vi "Test Server.vi"() -> ()   [LabVIEW 2013]
uses:
  <vilib>/LabVIEW Open Source Project/MQTT Control Packets/Control Packets/CONNACK/Connect Return Code -- enum.ctl
  Server/Server class/Server.lvclass/Server.ctl
  Client/Client Class/Client.lvclass/Client.ctl
  <vilib>/LabVIEW Open Source Project/MQTT Control Packets/Control Packets/PUBLISH/PUBLISH.lvclass
  Server/Server class/Server.lvclass
  MQTT_Base/Base Class/MQTT_Base.lvclass
  Client/Client Class/Client.lvclass
  MQTT_TCP/Connection/TCPConnection.lvclass
  <vilib>/LabVIEW Open Source Project/MQTT Control Packets/Control Packets/CONNACK/CONNACK.lvclass
panel:
  out "error server":errorcluster
  in  "Unsubscribe":bool
  in  "Subscribe":bool
  out "error client sink 2":errorcluster
  out "Random 2":dbl(graph)
  out "received 2":i32
  out "received timer 2":u32
  out "Client Status 2":T1=enum."Server Unavailable"
  out "published timer":u32
  out "received timer":u32
  out "received":i32
  out "published":i32
  out "Random":dbl(graph)
  out "Client Status":T1=enum."Server Unavailable"
  out "error client source":errorcluster
  out "NbConnections":u32
  out "error client sink 1":errorcluster
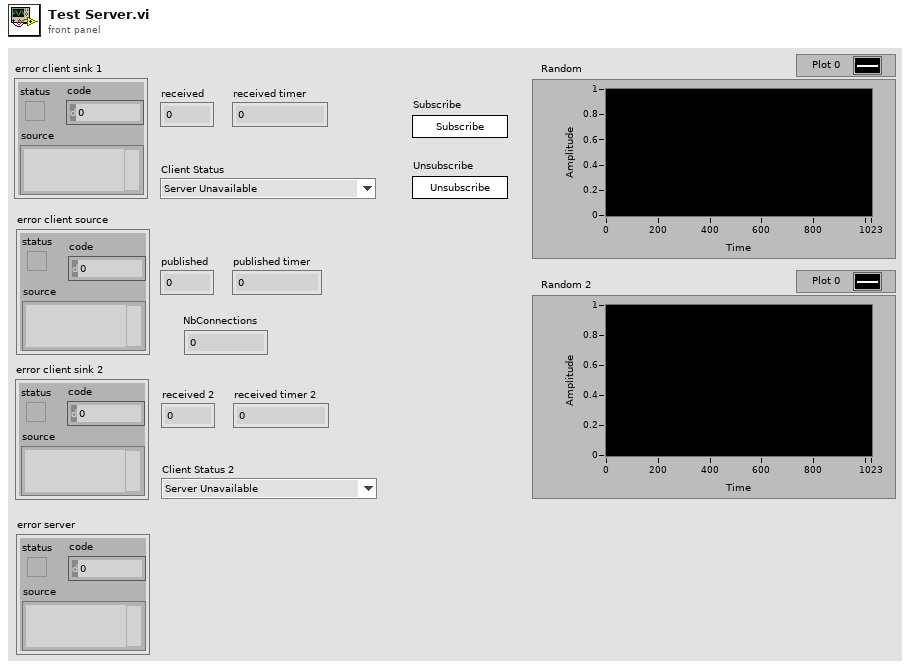
[diagram p1: front panel]
types:
  T1 = typedef "MQTT_Control_Packets.lvlib/CONNACK.lvclass/Connect Return Code -- enum.ctl" = enum16{"Connection accepted", "Unacceptable protocol version", "Identifier Rejected", "Server Unavailable", "Bad Username or Password", "Not Authorized"}
  T2 = typedef "MQTT Server.lvlib/Server.lvclass/Public Events -- cluster.ctl" = cluster{"NbConnections":refnum<user-event>}
  T3 = typedef "MQTT Client.lvlib/Client.lvclass/Public Events -- cluster.ctl" = cluster{"Connection Status":refnum<user-event>, "Connected":refnum<user-event>, "Application Message":refnum<user-event>}
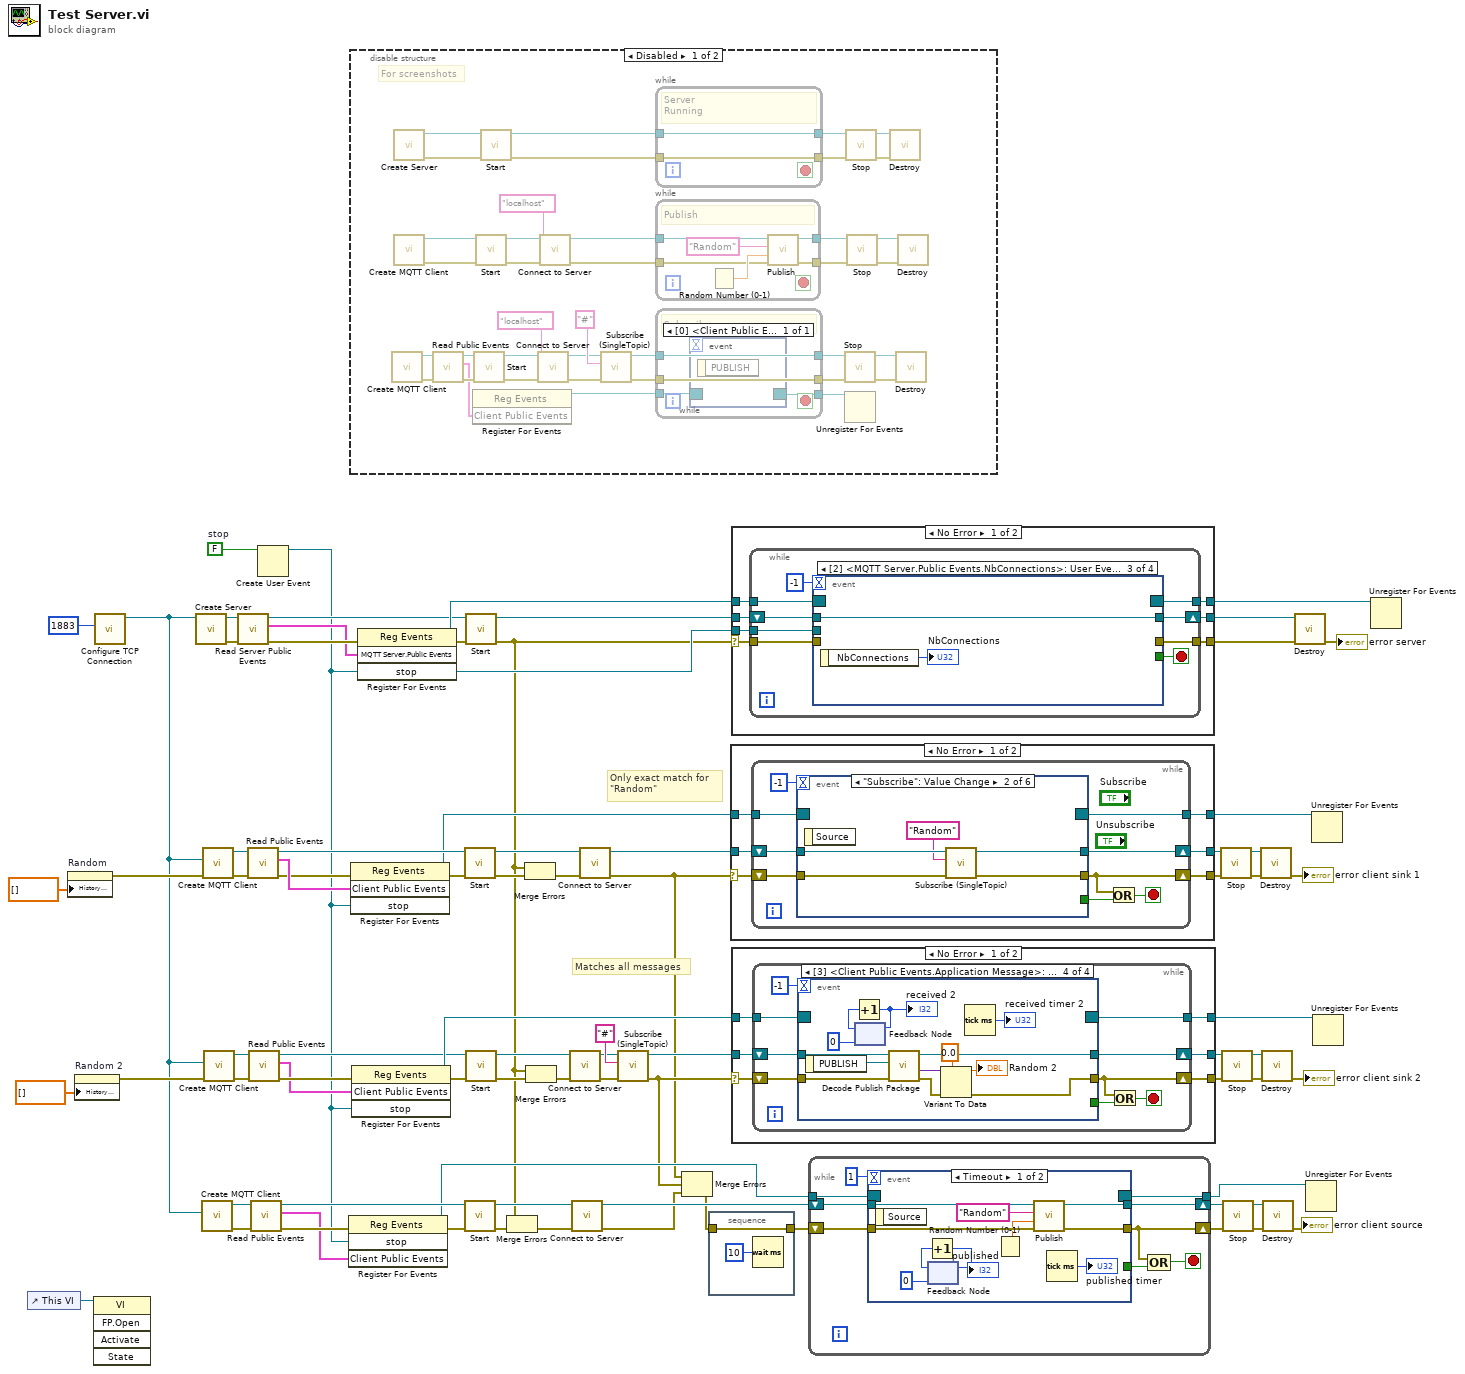
[diagram p0: block diagram]
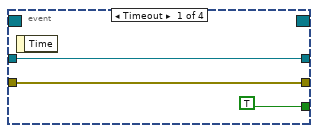
[diagram p3: hidden frame]
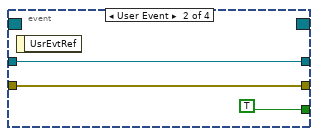
[diagram p4: hidden frame]
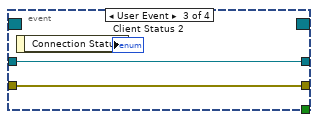
[diagram p5: hidden frame]
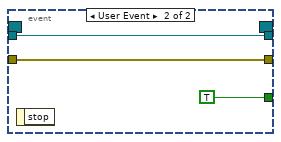
[diagram p7: hidden frame]
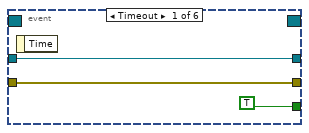
[diagram p8: hidden frame]
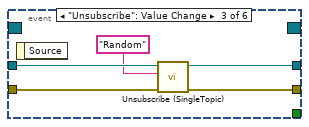
[diagram p9: hidden frame]
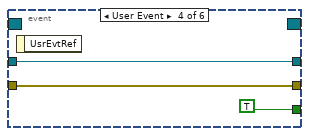
[diagram p10: hidden frame]
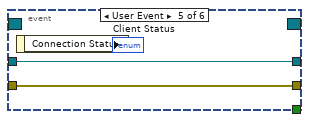
[diagram p11: hidden frame]
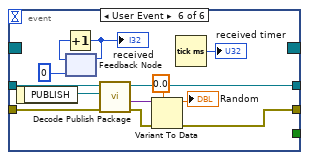
[diagram p12: hidden frame]
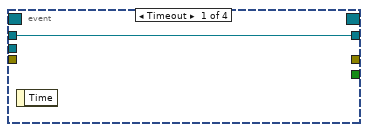
[diagram p14: hidden frame]
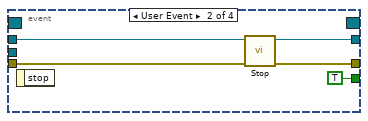
[diagram p15: hidden frame]
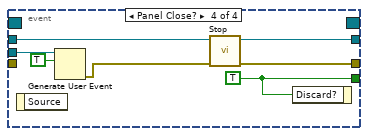
[diagram p16: hidden frame]
diagram:
  w39 = FALSE  # stop
  # "Matches all messages"
  # "Only exact match for\n\"Random\""
  n1 = control-ref of="This VI"() -> (w7:refnum<vi>)
  n2 = property on="Random" class="WFChart (strict)"("History Data"=dbl[] []) -> (error out=w43:errorcluster)  [unwired: 2 in, 1 out]
  n3 = property on="Random 2" class="WFChart (strict)"("History Data"=dbl[] []) -> (error out=w10:errorcluster)  [unwired: 2 in, 1 out]
  n4 = invoke class="VI" method="FP.Open"(reference=w7) -> ()  [unwired: 4 in, 5 out]
  n5 = call "Configure TCP Connection.vi"("remote port (80)"=u16 1883) -> ("TCPConnection"=w1:refnum<class "TCPConnection.lvclass">)  [unwired: 9 in, 1 out]
  n6 = call "Create Server.vi"("Connection Configuration"=w1) -> ("error out"=w79:errorcluster, "Server"=w80:refnum<class "Server.lvclass">)  [unwired: 9 in]
  n7 = call "Create MQTT Client.vi"("Connection Configuration"=w1) -> ("error out"=w63:errorcluster, "Client out"=w62:refnum<class "Client.lvclass">)  [unwired: 9 in]
  n8 = call "Create MQTT Client.vi"("error in (no error)"=w43, "Connection Configuration"=w1) -> ("error out"=w64:errorcluster, "Client out"=w65:refnum<class "Client.lvclass">)  [unwired: 8 in]
  n9 = call "Create MQTT Client.vi"("error in (no error)"=w10, "Connection Configuration"=w1) -> ("error out"=w15:errorcluster, "Client out"=w14:refnum<class "Client.lvclass">)  [unwired: 8 in]
  n10 = call "Read Server Public Events.vi"("error in (no error)"=w79, "Server in"=w80) -> ("error out"=w78:errorcluster, "MQTT Server.Public Events"=w77:T2, "Server out"=w73:refnum<class "Server.lvclass">)  [unwired: 7 in]
  n11 = call "Read Public Events.vi"("error in (no error)"=w64, "Client in"=w65) -> ("error out"=w48:errorcluster, "Client Public Events"=w49:T3, "Client out"=w61:refnum<class "Client.lvclass">)  [unwired: 7 in]
  n12 = call "Read Public Events.vi"("error in (no error)"=w15, "Client in"=w14) -> ("error out"=w26:errorcluster, "Client Public Events"=w25:T3, "Client out"=w16:refnum<class "Client.lvclass">)  [unwired: 7 in]
  n13 = call "Read Public Events.vi"("error in (no error)"=w63, "Client in"=w62) -> ("error out"=w38:errorcluster, "Client Public Events"=w34:T3, "Client out"=w58:refnum<class "Client.lvclass">)  [unwired: 7 in]
  n14 = Create User Event(user event datatype=w39) -> (user event=w11:refnum<user-event>)  [unwired: 1 in, 1 out]
  n15 = register-events(error in=w38, w11, w34) -> (reference out=w36:refnum<event-registration>, error out=w37:errorcluster)  [unwired: 1 in]
  n16 = disable-structure shown="Disabled" {
    frame Disabled {
      # "For screenshots"
      n17 = call "Create MQTT Client.vi"() -> ("error out"=w86:errorcluster, "Client out"=w88:refnum<class "Client.lvclass">)  [unwired: 10 in]
      n18 = call "Create Server.vi"() -> ("error out"=w113:errorcluster, "Server"=w112:refnum<class "Server.lvclass">)  [unwired: 10 in]
      n19 = call "Create MQTT Client.vi"() -> ("error out"=w110:errorcluster, "Client out"=w111:refnum<class "Client.lvclass">)  [unwired: 10 in]
      n20 = call "Read Public Events.vi"("error in (no error)"=w86, "Client in"=w88) -> ("error out"=w85:errorcluster, "Client Public Events"=w84:T3, "Client out"=w87:refnum<class "Client.lvclass">)  [unwired: 7 in]
      n21 = register-events(w84) -> (reference out=w83:refnum<event-registration>)  [unwired: 2 in, 1 out]
      n22 = call "Start.vi"("error in (no error)"=w85, "MQTT_Base in"=w87) -> ("error out"=w103:errorcluster, "MQTT_Base out"=w104:refnum<class "Client.lvclass">)  [unwired: 7 in, 1 out]
      n23 = call "Start.vi"("error in (no error)"=w110, "MQTT_Base in"=w111) -> ("error out"=w117:errorcluster, "MQTT_Base out"=w116:refnum<class "Client.lvclass">)  [unwired: 7 in, 1 out]
      n24 = call "Start.vi"("error in (no error)"=w113, "MQTT_Base in"=w112) -> ("error out"=w95:errorcluster, "MQTT_Base out"=w97:refnum<class "Server.lvclass">)  [unwired: 7 in, 1 out]
      n25 = call "Connect to Server.vi"("error in (no error)"=w103, 10:"localhost" ("Topic Filter"), "Client in"=w104) -> ("error out"=w91:errorcluster, "Client out"=w92:refnum<class "Client.lvclass">)  [unwired: 5 in, 2 out]
      n26 = call "Connect to Server.vi"("error in (no error)"=w117, 10:"localhost" ("Topic Filter"), "Client in"=w116) -> ("error out"=w99:errorcluster, "Client out"=w102:refnum<class "Client.lvclass">)  [unwired: 5 in, 2 out]
      n27 = call "Subscribe (SingleTopic).vi"("error in (no error)"=w91, "Topic Filter"="#", "MQTT_Base in"=w92) -> ("error out"=w89:errorcluster, "MQTT_Base out"=w90:refnum<class "Client.lvclass">)  [unwired: 7 in]
      n28 = while {
        tunnel: [w131] -> w98
        tunnel: w97 -> [w131]
        tunnel: w95 -> [w130]
        tunnel: [w130] -> w96
        stop <- _ stop-if-true
        # "Server\nRunning"
      }
      n29 = while {
        tunnel: w102 -> [w127]
        tunnel: [w126] -> w101
        tunnel: [w125] -> w100
        tunnel: w99 -> [w124]
        stop <- _ stop-if-true
        # "Publish"
        n30 = Random Number (0-1)() -> (number: 0 to 1=w129:dbl)
        n31 = call "Publish.vi"("error in (no error)"=w124, "Payload"=w129, "Topic Name (empty: Payload name)"="Random", "Client in"=w127) -> ("error out"=w125:errorcluster, "Client out"=w126:refnum<class "Client.lvclass">)  [unwired: 5 in, 1 out]
      }
      n32 = while {
        tunnel: [w123] -> w93
        tunnel: w90 -> [w123]
        tunnel: w89 -> [w122]
        tunnel: [w122] -> w94
        tunnel: w83 -> [w121]
        tunnel: [w120] -> w82
        stop <- _ stop-if-true
        # "Subscribe"
        n33 = event shown="[0] <Client Public Events.Application Message>: User Event" {
          selector: w121 -> [_]
          dyn-events: [_] -> w120
          timeout: _ -> [_]
          event User Event {
            n34 = event-data() -> ()  [unwired: 1 in, 1 out]
          }
        }
      }
      n35 = call "Stop.vi"("error in (no error)"=w94, "MQTT_Base in"=w93) -> ("error out"=w106:errorcluster, "MQTT_Base out"=w107:refnum<class "Client.lvclass">)  [unwired: 7 in, 1 out]
      n36 = Unregister For Events(event registration refnum=w82) -> ()  [unwired: 1 in, 1 out]
      n37 = call "Stop.vi"("error in (no error)"=w96, "MQTT_Base in"=w98) -> ("error out"=w119:errorcluster, "MQTT_Base out"=w118:refnum<class "Server.lvclass">)  [unwired: 7 in, 1 out]
      n38 = call "Stop.vi"("error in (no error)"=w100, "MQTT_Base in"=w101) -> ("error out"=w115:errorcluster, "MQTT_Base out"=w114:refnum<class "Client.lvclass">)  [unwired: 7 in, 1 out]
      n39 = call "Destroy.vi"("error in (no error)"=w119, "MQTT_Base in"=w118) -> ()  [unwired: 8 in, 2 out]
      n40 = call "Destroy.vi"("error in (no error)"=w106, "MQTT_Base in"=w107) -> ()  [unwired: 8 in, 2 out]
      n41 = call "Destroy.vi"("error in (no error)"=w115, "MQTT_Base in"=w114) -> ()  [unwired: 8 in, 2 out]
    }
    frame Enabled {
    }
  }
  n42 = register-events(error in=w48, w49, w11) -> (reference out=w46:refnum<event-registration>, error out=w47:errorcluster)  [unwired: 1 in]
  n43 = register-events(error in=w26, w25, w11) -> (reference out=w28:refnum<event-registration>, error out=w27:errorcluster)  [unwired: 1 in]
  n44 = register-events(error in=w78, w77, w11) -> (reference out=w76:refnum<event-registration>, error out=w71:errorcluster)  [unwired: 1 in]
  n45 = call "Start.vi"("error in (no error)"=w47, "MQTT_Base in"=w61) -> ("error out"=w59:errorcluster, "MQTT_Base out"=w60:refnum<class "Client.lvclass">)  [unwired: 7 in, 1 out]
  n46 = call "Start.vi"("error in (no error)"=w37, "MQTT_Base in"=w58) -> ("error out"=w56:errorcluster, "MQTT_Base out"=w57:refnum<class "Client.lvclass">)  [unwired: 7 in, 1 out]
  n47 = call "Start.vi"("error in (no error)"=w71, "MQTT_Base in"=w73) -> ("error out"=w9:errorcluster, "MQTT_Base out"=w72:refnum<class "Server.lvclass">)  [unwired: 7 in, 1 out]
  n48 = call "Start.vi"("error in (no error)"=w27, "MQTT_Base in"=w16) -> ("error out"=w18:errorcluster, "MQTT_Base out"=w17:refnum<class "Client.lvclass">)  [unwired: 7 in, 1 out]
  n49 = Merge Errors(w9, w56) -> (w66:errorcluster)
  n50 = Merge Errors(w9, w59) -> (w67:errorcluster)
  n51 = Merge Errors(w9, w18) -> (w13:errorcluster)
  n52 = call "Connect to Server.vi"("error in (no error)"=w13, "Client in"=w17) -> ("error out"=w22:errorcluster, "Client out"=w21:refnum<class "Client.lvclass">)  [unwired: 6 in, 2 out]
  n53 = call "Connect to Server.vi"("error in (no error)"=w66, "Client in"=w57) -> ("error out"=w33:errorcluster, "Client out"=w74:refnum<class "Client.lvclass">)  [unwired: 6 in, 2 out]
  n54 = call "Connect to Server.vi"("error in (no error)"=w67, "Client in"=w60) -> ("error out"=w4:errorcluster, "Client out"=w5:refnum<class "Client.lvclass">)  [unwired: 6 in, 2 out]
  n55 = call "Subscribe (SingleTopic).vi"("error in (no error)"=w22, "Topic Filter"="#", "MQTT_Base in"=w21) -> ("error out"=w8:errorcluster, "MQTT_Base out"=w30:refnum<class "Client.lvclass">)  [unwired: 7 in]
  n56 = Merge Errors(w4, w8, w33) -> (w41:errorcluster)
  n57 = stacked-sequence {
    tunnel: [w132] -> w40
    tunnel: w41 -> [w132]
    frame #0 {
      n58 = Wait (ms)(milliseconds to wait=u32 10) -> ()  [unwired: 1 out]
    }
  }
  n59 = case shown="No Error" w4 {
    selector: w4 -> [w134 w181]
    tunnel: w46 -> [w139 w183]
    tunnel: [w138 w183] -> w45
    tunnel: w5 -> [w137 w182]
    tunnel: [w136 w182] -> w44
    tunnel: [w135 w181] -> w42
    frame No Error {
      n60 = while {
        tunnel: w139 -> [w148]
        tunnel: [w147] -> w138
        shift-right: [w145] -> w136
        shift-left: w137 -> [w146]
        shift-right: [w142] -> w135
        shift-left: w134 -> [w144]
        stop <- w143 stop-if-true
        n61 = event shown="[1] \"Subscribe\": Value Change" {
          selector: w148 -> [_ _ _ _ _ _]
          dyn-events: [_ _ _ _ _ _] -> w147
          timeout: -1 -> [_ _ _ _ _ _]
          tunnel: w146 -> [w150 w156 w161 w163 w166 w179]
          tunnel: [w150 w153 w160 w163 w166 w175] -> w145
          tunnel: [w149 w152 w157 w162 w165 w168] -> w142
          tunnel: w144 -> [w149 w155 w158 w162 w165 w174]
          tunnel: [TRUE _ _ TRUE _ _] -> w141
          event Timeout {
            n62 = event-data() -> ()  [unwired: 1 in, 1 out]
          }
          event "Subscribe": Value Change {
            n63 = event-data() -> ()  [unwired: 1 in, 1 out]
            n64 = call "Subscribe (SingleTopic).vi"("error in (no error)"=w155, "Topic Filter"="Random", "MQTT_Base in"=w156) -> ("error out"=w152:errorcluster, "MQTT_Base out"=w153:refnum<class "Client.lvclass">)  [unwired: 7 in]
          }
          event "Unsubscribe": Value Change {
            n65 = event-data() -> ()  [unwired: 1 in, 1 out]
            n66 = call "Unsubscribe (SingleTopic).vi"("error in (no error)"=w158, "Topic Filter"="Random", "MQTT_Base in"=w161) -> ("error out"=w157:errorcluster, "MQTT_Base out"=w160:refnum<class "Client.lvclass">)  [unwired: 7 in]
          }
          event User Event {
            n67 = event-data() -> ()  [unwired: 1 in, 1 out]
          }
          event User Event {
            n68 = event-data() -> ("Connection Status"=→"Client Status":T1)  [unwired: 1 in]
          }
          event User Event {
            n69 = event-data() -> ("PUBLISH"=w180:refnum<class "PUBLISH.lvclass">)  [unwired: 1 in]
            n70 = feedback #1(0 ("received")) -> (w172:i32)
            n71 = Increment(x=w172) -> (x+1=w171:i32)
            "received" <- w171
            n72 = feedback-in #1(w171) -> ()
            n73 = call "Decode Publish Package.vi"("error in (no error)"=w174, "PUBLISH in"=w180, "MQTT_Base in"=w179) -> ("error out"=w169:errorcluster, "Payload"=w178:variant, "MQTT_Base out"=w175:refnum<class "Client.lvclass">)  [unwired: 5 in, 1 out]
            n74 = Variant To Data(error in=w169, type=0.0, Variant=w178) -> (data=→"Random":dbl, error out=w168:errorcluster)
            n75 = Tick Count (ms)() -> (millisecond timer value=→"received timer":u32)
          }
        }
        n76 = Or(x=w142, y=w141) -> (x .or. y?=w143:bool)
      }
    }
    frame Error {
    }
  }
  n77 = case shown="No Error" w9 {
    selector: w9 -> [w184 w215]
    tunnel: w72 -> [w190 w217]
    tunnel: [w189 w217] -> w81
    tunnel: w76 -> [w188 w216]
    tunnel: [w187 w216] -> w75
    tunnel: [w186 w215] -> w70
    tunnel: w11 -> [w185 _]
    frame No Error {
      n78 = while {
        shift-right: [w196] -> w189
        shift-left: w190 -> [w198]
        tunnel: w188 -> [w195]
        tunnel: [w194] -> w187
        tunnel: [w193] -> w186
        tunnel: w185 -> [w192]
        tunnel: w184 -> [w191]
        stop <- w197 stop-if-true
        n79 = event shown="[2] <MQTT Server.Public Events.NbConnections>: User Event" {
          selector: w195 -> [_ _ _ _]
          dyn-events: [_ _ _ _] -> w194
          timeout: -1 -> [_ _ _ _]
          tunnel: w198 -> [w200 w205 w207 w214]
          tunnel: [_ TRUE ("Discard?") _ w213] -> w197
          tunnel: [w200 w204 w207 w212] -> w196
          tunnel: [_ w203 _ w211] -> w193
          tunnel: w192 -> [_ _ _ w210]
          tunnel: w191 -> [_ w201 _ _]
          event Timeout {
            n80 = event-data() -> ()  [unwired: 1 in, 1 out]
          }
          event User Event {
            n81 = event-data() -> ()  [unwired: 1 in, 1 out]
            n82 = call "Stop.vi"("error in (no error)"=w201, "MQTT_Base in"=w205) -> ("error out"=w203:errorcluster, "MQTT_Base out"=w204:refnum<class "Server.lvclass">)  [unwired: 7 in, 1 out]
          }
          event User Event {
            n83 = event-data() -> ("NbConnections"=→"NbConnections":u32)  [unwired: 1 in]
          }
          event Panel Close? {
            w213 = TRUE ("Discard?")
            n84 = event-data() -> ()  [unwired: 1 in, 1 out]
            n85 = Generate User Event(user event=w210, event data cluster=TRUE ("event data")) -> (error out=w208:errorcluster)  [unwired: 2 in, 1 out]
            n86 = call "Stop.vi"("error in (no error)"=w208, "MQTT_Base in"=w214) -> ("error out"=w211:errorcluster, "MQTT_Base out"=w212:refnum<class "Server.lvclass">)  [unwired: 7 in, 1 out]
            n87 = event-data("Discard?"=w213) -> ()  [unwired: 1 in, 1 out]
          }
        }
      }
    }
    frame Error {
    }
  }
  n88 = case shown="No Error" w8 {
    selector: w8 -> [w218 w255]
    tunnel: w28 -> [w223 w257]
    tunnel: [w222 w257] -> w29
    tunnel: w30 -> [w221 w256]
    tunnel: [w220 w256] -> w31
    tunnel: [w219 w255] -> w32
    frame No Error {
      n89 = while {
        tunnel: w223 -> [w232]
        tunnel: [w231] -> w222
        shift-right: [w229] -> w220
        shift-left: w221 -> [w230]
        shift-right: [w226] -> w219
        shift-left: w218 -> [w228]
        stop <- w227 stop-if-true
        n90 = event shown="[3] <Client Public Events.Application Message>: User Event" {
          selector: w232 -> [_ _ _ _]
          dyn-events: [_ _ _ _] -> w231
          timeout: -1 -> [_ _ _ _]
          tunnel: w230 -> [w234 w237 w240 w253]
          tunnel: [w234 w237 w240 w249] -> w229
          tunnel: [w233 w236 w239 w242] -> w226
          tunnel: w228 -> [w233 w236 w239 w248]
          tunnel: [TRUE TRUE _ _] -> w225
          event Timeout {
            n91 = event-data() -> ()  [unwired: 1 in, 1 out]
          }
          event User Event {
            n92 = event-data() -> ()  [unwired: 1 in, 1 out]
          }
          event User Event {
            n93 = event-data() -> ("Connection Status"=→"Client Status 2":T1)  [unwired: 1 in]
          }
          event User Event {
            n94 = event-data() -> ("PUBLISH"=w254:refnum<class "PUBLISH.lvclass">)  [unwired: 1 in]
            n95 = feedback #2(0 ("received")) -> (w246:i32)
            n96 = Increment(x=w246) -> (x+1=w245:i32)
            "received 2" <- w245
            n97 = feedback-in #2(w245) -> ()
            n98 = call "Decode Publish Package.vi"("error in (no error)"=w248, "PUBLISH in"=w254, "MQTT_Base in"=w253) -> ("error out"=w243:errorcluster, "Payload"=w252:variant, "MQTT_Base out"=w249:refnum<class "Client.lvclass">)  [unwired: 5 in, 1 out]
            n99 = Variant To Data(error in=w243, type=0.0, Variant=w252) -> (data=→"Random 2":dbl, error out=w242:errorcluster)
            n100 = Tick Count (ms)() -> (millisecond timer value=→"received timer 2":u32)
          }
        }
        n101 = Or(x=w226, y=w225) -> (x .or. y?=w227:bool)
      }
    }
    frame Error {
    }
  }
  n102 = while {
    shift-right: [w265] -> w55
    shift-left: w74 -> [w266]
    shift-right: [w263] -> w35
    shift-left: w40 -> [w264]
    tunnel: w36 -> [w261]
    tunnel: [w259] -> w6
    stop <- w262 stop-if-true
    n103 = event shown="[0] Timeout" {
      selector: w261 -> [_ _]
      dyn-events: [_ _] -> w259
      timeout: 1 -> [_ _]
      tunnel: w266 -> [w272 w277]
      tunnel: [w271 w277] -> w265
      tunnel: w264 -> [w270 w278]
      tunnel: [w269 w278] -> w263
      tunnel: [_ TRUE] -> w260
      event Timeout {
        n104 = event-data() -> ()  [unwired: 1 in, 1 out]
        n105 = feedback #3(0 ("received")) -> (w275:i32)
        n106 = Increment(x=w275) -> (x+1=w273:i32)
        "published" <- w273
        n107 = feedback-in #3(w273) -> ()
        n108 = Random Number (0-1)() -> (number: 0 to 1=w267:dbl)
        n109 = call "Publish.vi"("error in (no error)"=w270, "Payload"=w267, "Topic Name (empty: Payload name)"="Random", "Client in"=w272) -> ("error out"=w269:errorcluster, "Client out"=w271:refnum<class "Client.lvclass">)  [unwired: 5 in, 1 out]
        n110 = Tick Count (ms)() -> (millisecond timer value=→"published timer":u32)
      }
      event User Event {
        n111 = event-data() -> ()  [unwired: 1 in, 1 out]
      }
    }
    n112 = Compound Arithmetic op=OR(w263, w260) -> (w262:bool)
  }
  n113 = call "Stop.vi"("error in (no error)"=w42, "MQTT_Base in"=w44) -> ("error out"=w52:errorcluster, "MQTT_Base out"=w51:refnum<class "Client.lvclass">)  [unwired: 7 in, 1 out]
  n114 = call "Stop.vi"("error in (no error)"=w32, "MQTT_Base in"=w31) -> ("error out"=w19:errorcluster, "MQTT_Base out"=w20:refnum<class "Client.lvclass">)  [unwired: 7 in, 1 out]
  n115 = call "Stop.vi"("error in (no error)"=w35, "MQTT_Base in"=w55) -> ("error out"=w53:errorcluster, "MQTT_Base out"=w54:refnum<class "Client.lvclass">)  [unwired: 7 in, 1 out]
  n116 = call "Destroy.vi"("error in (no error)"=w52, "MQTT_Base in"=w51) -> ("error out"=→"error client sink 1":errorcluster)  [unwired: 8 in, 1 out]
  n117 = call "Destroy.vi"("error in (no error)"=w19, "MQTT_Base in"=w20) -> ("error out"=→"error client sink 2":errorcluster)  [unwired: 8 in, 1 out]
  n118 = call "Destroy.vi"("error in (no error)"=w53, "MQTT_Base in"=w54) -> ("error out"=→"error client source":errorcluster)  [unwired: 8 in, 1 out]
  n119 = call "Destroy.vi"("error in (no error)"=w70, "MQTT_Base in"=w81) -> ("error out"=→"error server":errorcluster)  [unwired: 8 in, 1 out]
  n120 = Unregister For Events(event registration refnum=w6) -> ()  [unwired: 1 in, 1 out]
  n121 = Unregister For Events(event registration refnum=w45) -> ()  [unwired: 1 in, 1 out]
  n122 = Unregister For Events(event registration refnum=w29) -> ()  [unwired: 1 in, 1 out]
  n123 = Unregister For Events(event registration refnum=w75) -> ()  [unwired: 1 in, 1 out]
